vi "Initialize Front Panel.vi"(8 "error in (no error)":errorcluster, 11 "BoundViewManager in":refnum<class "BoundViewManager.lvclass">) -> (0 "error out":errorcluster, 3 "BoundViewManager out":refnum<class "BoundViewManager.lvclass">)   [LabVIEW 2015, in "BoundViewManager.lvlib" / "BoundViewManager.lvclass"]
doc: "<License>\nCopyright © 2017 Composed Systems, LLC | All rights reserved\nwww.composed.io\n\nAuthor: Ethan Stern <ethan.stern@composed.io>\n\nThis software is provided \"AS IS\" WITHOUT WARRANTIES, either express or implied, AND IS FOR EDUCATIONAL PURPOSES ONLY.\n</License>"
uses:
  BoundViewManager.lvclass
  BoundViewManager.lvclass/BoundViewManager.ctl
  <vilib>/ActorFramework/Message Enqueuer/Message Enqueuer.lvclass
  Framework/IViewable/IViewable Messages/Insert Front Panel Msg/Insert Front Panel Msg.lvclass/Insert Front Panel Msg.ctl
  <vilib>/ActorFramework/Message Enqueuer/Message Enqueuer.lvclass/Message Enqueuer.ctl
  <vilib>/ActorFramework/Message Enqueuer/Enqueue.vi
  <vilib>/ActorFramework/Message Priority Queue/Priority Enqueue.vi
  Framework/IViewManager/IViewManager/IViewManager.lvclass
  Framework/IViewable/IViewable Messages/Insert Front Panel Msg/Insert Front Panel Msg.lvclass
  <vilib>/Composed Systems/Current Value Table/CurrentValueTable.lvclass
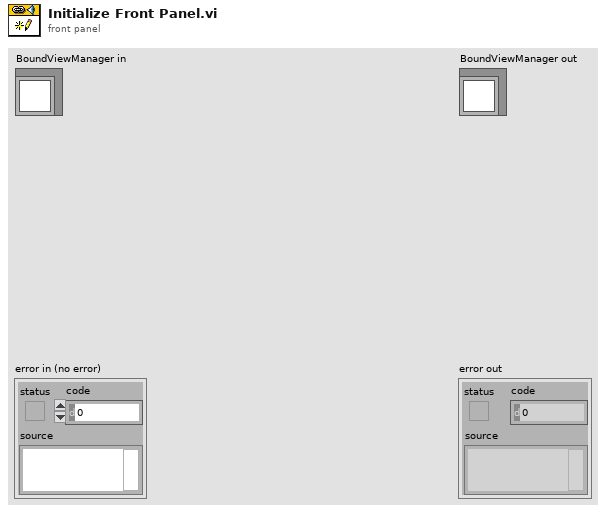
[diagram p1: front panel]
types:
  T1 = typedef "CurrentValueTable.lvlib/CurrentValueTable.lvclass/CurrentValueTable Reference.ctl" = refnum<data-value>
  T2 = typedef "IViewable.lvlib/ProtectedSubpanel.lvclass/Protected Subpanel Reference.ctl" = refnum<data-value>
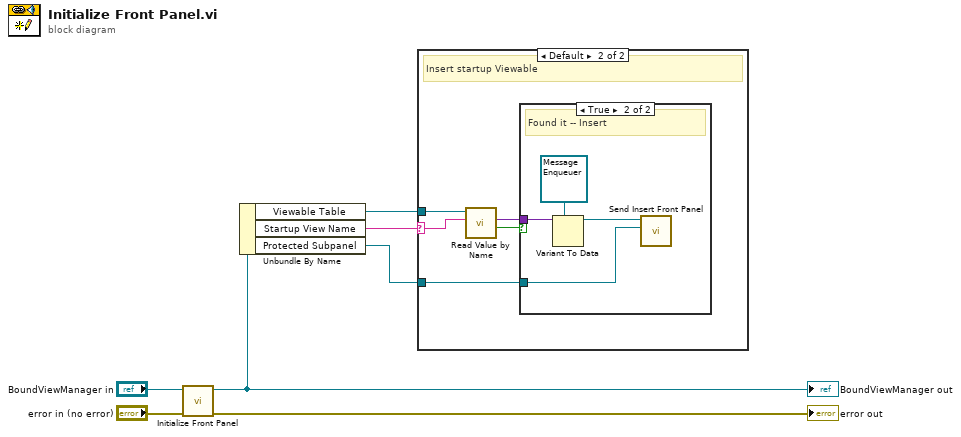
[diagram p0: block diagram]
diagram:
  n1 = call-parent "Initialize Front Panel.vi"("error in (no error)"="error in (no error)", "IViewable in"="BoundViewManager in") -> ("error out"=→"error out":errorcluster, "IViewable out"=w4:refnum<class "BoundViewManager.lvclass">)  [unwired: 8 in]
  "BoundViewManager out" <- w4
  n2 = Unbundle By Name(w4) -> ("Viewable Table"=w2:T1, "Startup View Name"=w3:string, "Protected Subpanel"=w1:T2)
  n3 = case shown="Default" w3 {
    selector: w3 -> [_ w11]
    tunnel: w2 -> [_ w12]
    tunnel: w1 -> [_ w8]
    frame "" {
      # "No startup viewable insertion"
    }
    frame Default {
      # "Insert startup Viewable"
      n4 = call <vilib>:"Read Value by Name.vi"("Data Name"=w11, "Current Value Table"=w12) -> ("Value Found?"=w10:bool, "Current Value"=w9:variant)  [unwired: 6 in, 2 out]
      n5 = case shown="True" w10 {
        tunnel: w9 -> [_ w16]
        tunnel: w8 -> [_ w13]
        frame False {
          # "Not found"
        }
        frame True {
          # "Found it -- Insert"
          n6 = Variant To Data(type=refnum<class "Message Enqueuer.lvclass"> refnum ("Message Enqueuer"), Variant=w16) -> (data=w14:refnum<class "Message Enqueuer.lvclass">)  [unwired: 1 in, 1 out]
          n7 = call "Send Insert Front Panel.vi"("Protected Subpanel"=w13, "Message Enqueuer"=w14) -> ()  [unwired: 8 in, 2 out]
        }
      }
    }
  }
